vi "dOD array to waveform.vi"(7 "DAQ":T1={"Input Config"=10106, "Card"=enum."USB-6251", "100% Reflectance Standard (V)"=1.0, "Input Channel"="Dev1/ai0", "Final number of points"=0.0, "Average number of points"=1.0, "Number of samples"=10000.0, "Trigger Level (V)"=0.2, "Rate"=1250000, "End Time (s)"=0.05, "dt"=5e-06, "time array (decimated)"=[], "DOD (final)"=[], "Live data"={"t0"=timestamp(0 s since 1904-01-01), "dt"=1.0, "Y"=[]}, "DAQ task"="", "Max number of shots (to match scope)"=0, "data array"=[], "Last state"=enum."Start", "Shot counter"=10, "Test counter"=0, "Averaged data"={"t0"=timestamp(0 s since 1904-01-01), "dt"=1.0, "Y"=[]}, "Background level (V)"=0.0} {"Input Config" items=["default"=-1, "RSE"=10083, "NRSE"=10078, "Differential"=10106, "Pseudodifferential"=12529]}, 11 "Y array":dbl[](array[numeric])) -> (3 "waveform":waveform(dbl))   [LabVIEW 2017, in "Processing.lvlib"]
uses:
  Controls/Params.ctl
  Controls/Commands [enum].ctl
  Processing/Processing.lvlib
  DAQ.lvlib
panel:
  # "indicators"
  # "internal use"
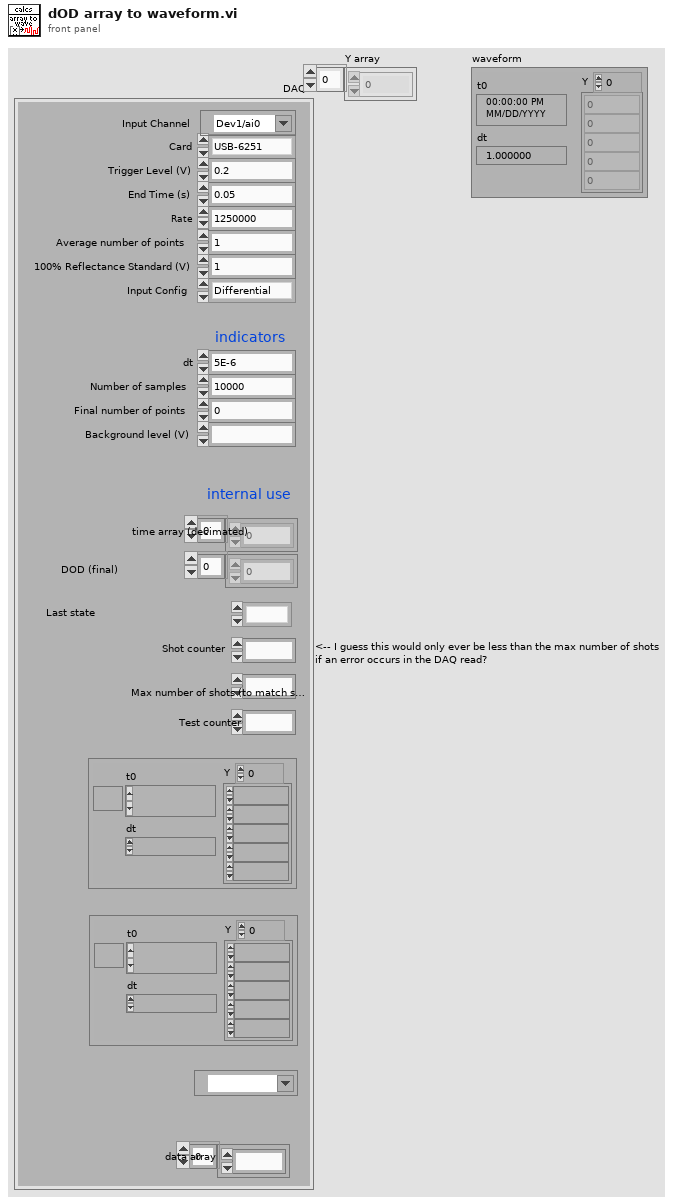
[diagram p1: front panel]
types:
  T1 = typedef "DAQ.lvlib/Params.ctl" = cluster{"Input Config":i32, "Card":enum16{"USB-6211", "USB-6251"}, "100% Reflectance Standard (V)":dbl, "Input Channel":tag, "Final number of points":dbl, "Average number of points":dbl, "Number of samples":dbl, "Trigger Level (V)":dbl, "Rate":i32, "End Time (s)":dbl, "dt":dbl, "time array (decimated)":dbl[], "DOD (final)":dbl[], "Live data":waveform(dbl), "DAQ task":refnum<k21>, "Max number of shots (to match scope)":i32, "data array":dbl[], "Last state":T2, "Shot counter":i32, "Test counter":i32, "Averaged data":waveform(dbl), "Background level (V)":dbl}
  T2 = typedef "DAQ.lvlib/Commands [enum].ctl" = enum16{"Start", "Stop", "Send data", "Get test data", "Accumulate test data", "Average test data", "Calculate background voltage"}
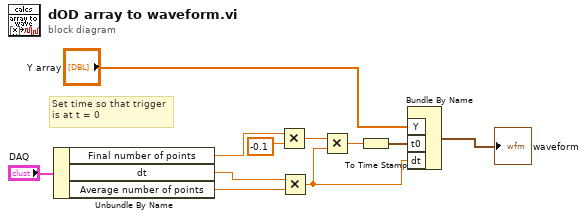
[diagram p0: block diagram]
diagram:
  # "Set time so that trigger\nis at t = 0"
  n1 = Unbundle By Name("DAQ") -> ("Final number of points"=w11:dbl, "dt"=w4:dbl, "Average number of points"=w3:dbl)
  n2 = Multiply(x=w11, y=-0.1) -> (x*y=w10:dbl)
  n3 = Multiply(x=w4, y=w3) -> (x*y=w8:dbl)
  n4 = Multiply(x=w10, y=w8) -> (x*y=w5:dbl)
  n5 = To Time Stamp(1:w5) -> (0:w9:timestamp)
  n6 = Bundle By Name("Y"="Y array", "t0"=w9, "dt"=w8) -> (→"waveform":waveform(dbl))  [unwired: 1 in]
